vi "MonitoringRetest.vi"() -> ()   [LabVIEW 2013]
panel:
  in  "Envoi":bool
  in  "data in":string
  out "?":bool
  in  "Afficher caractères reçus":bool
  in  "Log":bool
  out "error out":errorcluster
  out "Caractères reçus":string
  in  "Mode":T1(ring)=enum."CRLF"
  in  "?":bool
  in  "Tab Control":T2(tab)
  out "Signal Camera     ->    Fronts détectés":dbl[](graph)
  out "Signal Camera    ->  original":dbl[](graph)
  out "Moyenne":dbl
  out "Vitesse roue arrière gauche [m/s]":dbl(knob) scale=0.0..10.0
  out "Consigne gauche":dbl
  out "Effective gauche":dbl
  out "Vitesse roue arrière droite [m/s]":dbl(knob) scale=0.0..10.0
  out "Consigne droite":dbl
  out "Effective droite":dbl
  out "Position Servo":dbl(knob) scale=0.0..10.0
  out "?":dbl
  in  "PID 3.3":dbl
  in  "PID 3.2":dbl
  in  "PID Direction":dbl
  in  "ABS":bool
  out "?":bool
  in  "PID vitesse":bool
  out "?":bool
  out "?":bool
  in  "PID 2.3":i8
  in  "PID 2.2":i8
  in  "PID Léger":i8
  in  "PID 1.3":i8
  in  "PID 1.2":i8
  in  "PID Fort":i8
  out "Array":bool[](array[boolean])
  # "Fort"
  # "Léger"
  # "Droite"
  # "Gauche"
  # "Fin"
  # "Perte Ligne"
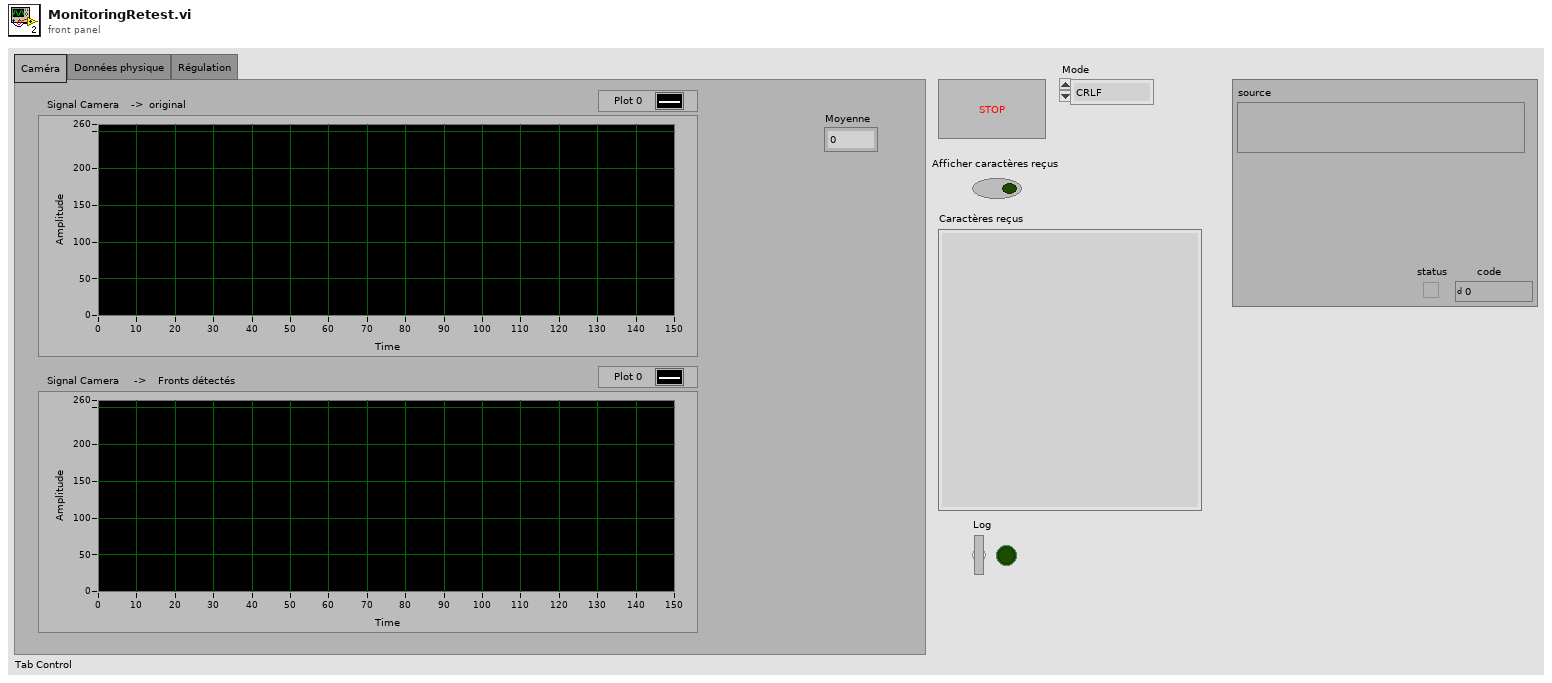
[diagram p1: front panel]
types:
  T1 = enum16{"Standard", "Buffered", "CRLF", "Immediate"}
  T2 = enum32{"Caméra", "Données physique", "Régulation"}
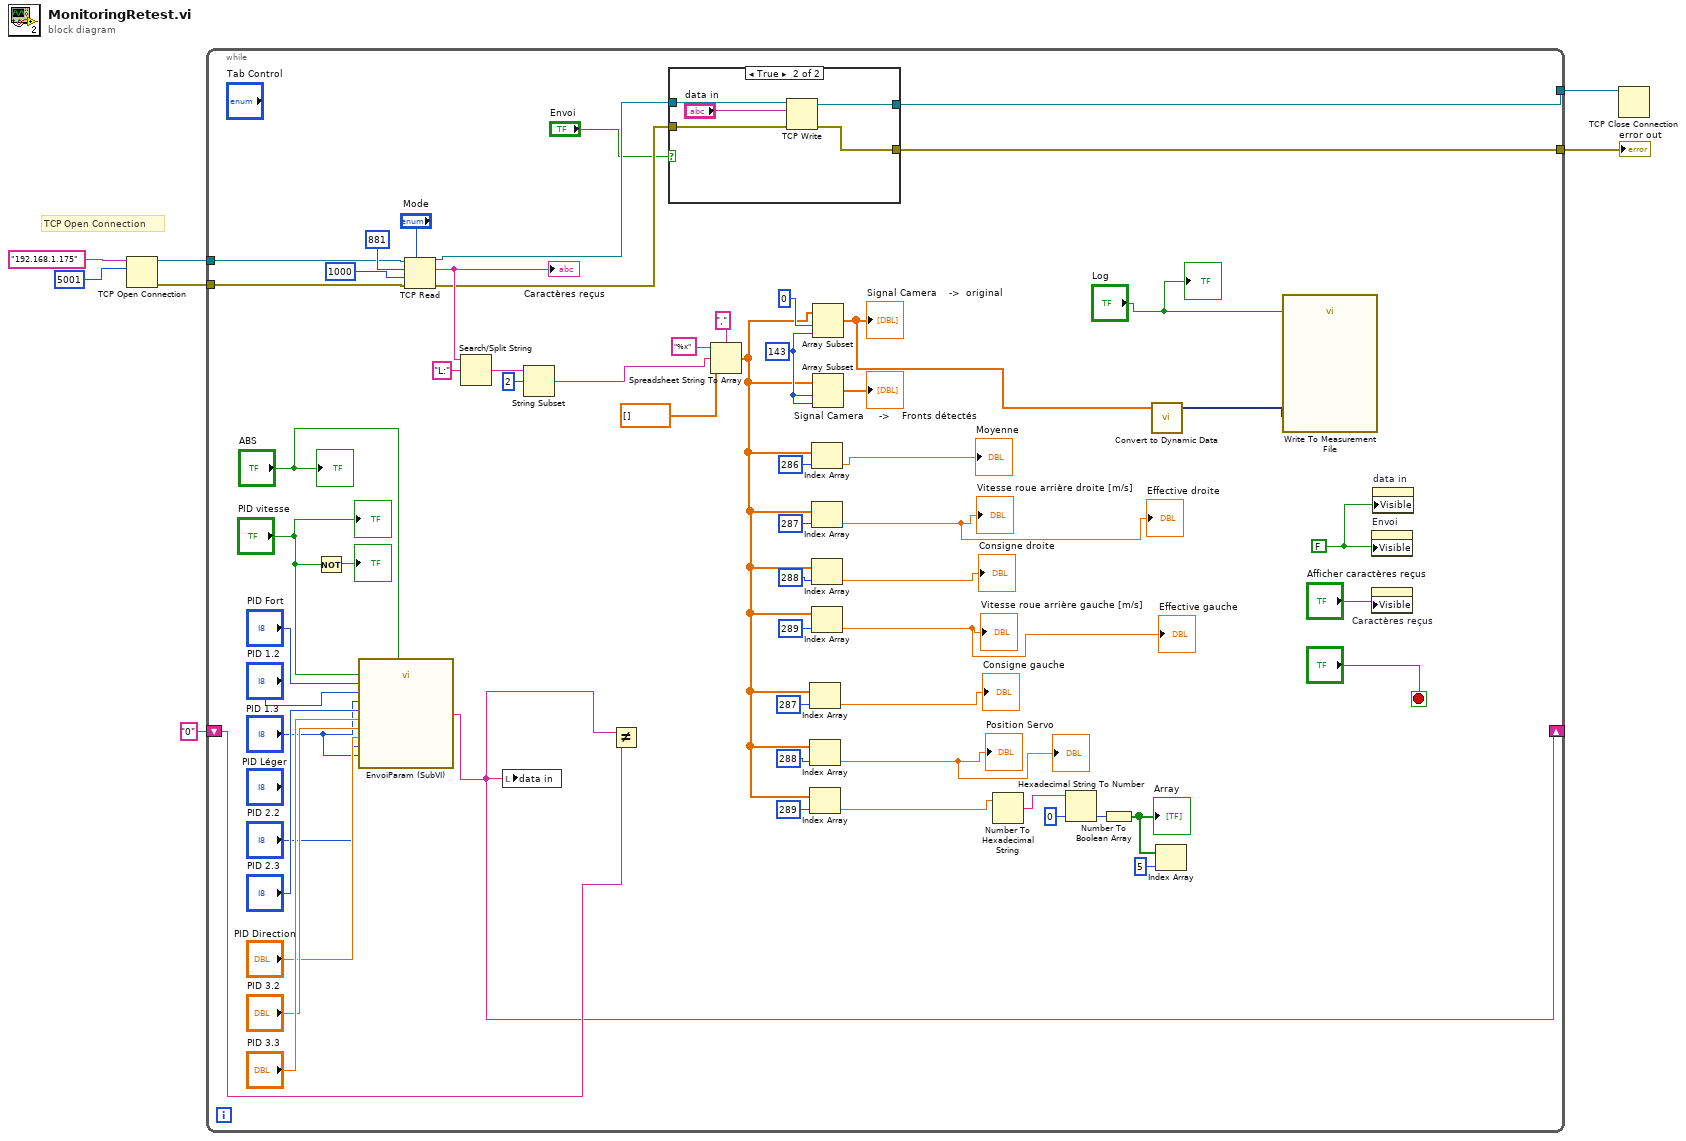
[diagram p0: block diagram]
diagram:
  # "TCP Open Connection"
  n1 = TCP Open Connection(address="192.168.1.175", remote port or service name=u16 5001) -> (connection ID=w5:refnum<k5>, error out=w4:errorcluster)  [unwired: 3 in]
  n2 = while {
    tunnel: w5 -> [w47]
    tunnel: w4 -> [w54]
    tunnel: [w45] -> w3
    tunnel: [w43] -> w2
    shift-right: [w30] -> _
    shift-left: "0" -> [w40]
    stop <- "?" stop-if-true
    w41 = FALSE
    w53 = 143 ("length")
    n3 = Not(x="PID vitesse") -> (.not. x?=→"?":bool)
    n4 = call "EnvoiParam (SubVI).vi"("PID 3.3"="PID 3.3", "PID 3.2"="PID 3.2", "PID Direction"="PID Direction", "PID 2.3"="PID 2.3", "PID 2.2"="PID 2.2", "PID Léger"="PID 1.3", "PID 1.3"="PID 1.3", "PID 1.2"="PID 1.2", "PID Fort"="PID Fort", "PID vitesse"="PID vitesse", "ABS"="ABS") -> ("String"=w30:string)
    n5 = TCP Read(connection ID=w47, bytes to read=881, error in (no error)=w54, 7:"Mode", 9:1000 ("timeout ms (25000)")) -> (connection ID out=w46:refnum<k5>, data out=w62:string, error out=w44:errorcluster)
    "Caractères reçus" <- w62
    n6 = Search/Split String(string=w62, search string/char (-)="L:") -> (match + rest of string=w60:string)  [unwired: 1 in, 2 out]
    n7 = local write "data in"(w30) -> ()
    n8 = String Subset(string=w60, offset (0)=2) -> (substring=w61:string)  [unwired: 1 in]
    n9 = Not Equal?(x=w30, y=w40) -> ()  [unwired: 1 out]
    n10 = case shown="True" "Envoi" {
      tunnel: w46 -> [w69 w74]
      tunnel: [w69 w73] -> w45
      tunnel: w44 -> [w68 w72]
      tunnel: [w68 w71] -> w43
      frame False {
      }
      frame True {
        n11 = TCP Write(connection ID=w74, data in="data in", error in (no error)=w72) -> (connection ID out=w73:refnum<k5>, error out=w71:errorcluster)  [unwired: 1 in, 1 out]
      }
    }
    n12 = Spreadsheet String To Array(delimiter (Tab)=",", format string="%x", spreadsheet string=w61, array type (2D Dbl)=dbl[] []) -> (array=w20:dbl[])
    n13 = Index Array(array=w20, index=287) -> (element=→"Consigne gauche":dbl)
    n14 = Index Array(array=w20, index=288) -> (element=→"Position Servo" →"?":dbl)
    n15 = Index Array(array=w20, index=289) -> (element=w11:dbl)
    n16 = Index Array(array=w20, index=286) -> (element=→"Moyenne":dbl)
    n17 = Index Array(array=w20, index=287) -> (element=→"Effective droite" →"Vitesse roue arrière droite [m/s]":dbl)
    n18 = Index Array(array=w20, index=288) -> (element=→"Consigne droite":dbl)
    n19 = Index Array(array=w20, index=289) -> (element=→"Vitesse roue arrière gauche [m/s]" →"Effective gauche":dbl)
    n20 = Array Subset(array=w20, index=0, length=w53) -> (w52:dbl[])
    "Signal Camera    ->  original" <- w52
    n21 = Array Subset(array=w20, index=w53, length=w53) -> (→"Signal Camera     ->    Fronts détectés":dbl[])
    n22 = Number To Hexadecimal String(2:w11) -> (0:w17:string)  [unwired: 1 in]
    n23 = Hexadecimal String To Number(string=w17, default (0uL)=u8 0 ("default (0 U32)")) -> (number=w18:u8)  [unwired: 1 in, 1 out]
    n24 = Number To Boolean Array(number=w18) -> (Boolean array=w16:bool[])
    "Array" <- w16
    n25 = call "Convert to Dynamic Data"("Array"=w52) -> ("Dynamic Data Type"=w50:dynamicdata)  [unwired: 3 in]
    n26 = Index Array(array=w16, index=5) -> ()  [unwired: 1 out]
    n27 = call "Write To Measurement File"("Signals"=w50, "Enable"="Log") -> ()  [unwired: 15 in, 3 out]
    n28 = property on="Envoi" class="Bool (strict)"("Visible"=w41) -> ()  [unwired: 2 in, 2 out]
    n29 = property on="Caractères reçus" class="Str"("Visible"="Afficher caractères reçus") -> ()  [unwired: 2 in, 2 out]
    n30 = property on="data in" class="Str"("Visible"=w41) -> ()  [unwired: 2 in, 2 out]
    "?" <- "ABS"
    "?" <- "PID vitesse"
    "?" <- "Log"
  }
  "error out" <- w2
  n31 = TCP Close Connection(connection ID=w3) -> ()  [unwired: 2 in, 2 out]
